vi "Read Position.vi"(8 "error in (no error)":errorcluster, 11 "Stage Actor.lvlib:Stage.lvclass":refnum<class "Stage.lvclass">) -> (0 "error out":errorcluster, 3 "Stage Actor.lvlib:Stage.lvclass":refnum<class "Stage.lvclass">)   [LabVIEW 2018, in "Stage Actor.lvlib" / "Stage.lvclass"]
uses:
  Stage.lvclass
  Stage.lvclass/Stage.ctl
  <instrlib>/Zaber A Series/Zaber A Series.lvlib
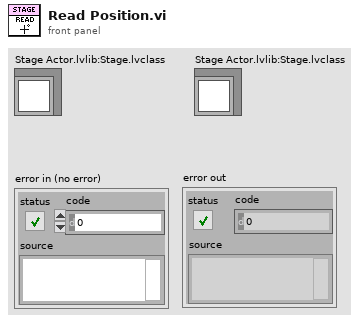
[diagram p1: front panel]
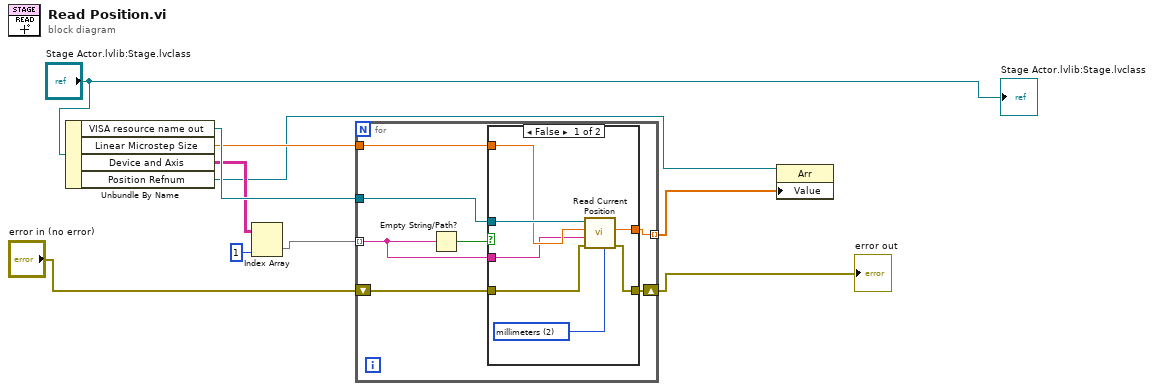
[diagram p0: block diagram]
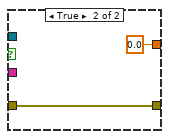
[diagram p2: hidden frame]
diagram:
  n1 = Unbundle By Name("Stage Actor.lvlib:Stage.lvclass") -> ("VISA resource name out"=w10:refnum<visa-resource-name>, "Linear Microstep Size"=w7:dbl, "Device and Axis"=w6:string[][], "Position Refnum"=w3:refnum<vi>)
  n2 = Index Array(array=w6, index (col)=1 ("disabled index (col)")) -> (element=w4:string[])  [unwired: 1 in]
  n3 = for {
    shift-right: [w16] -> w8
    shift-left: "error in (no error)" -> [w17]
    tunnel: [w14] -> w2 mode=indexing
    tunnel: w10 -> [w15]
    tunnel: w7 -> [w13]
    tunnel: w4 -> [w11] mode=indexing
    n4 = Empty String/Path?(string/path=w11) -> (empty?=w12:bool)
    n5 = case shown="False" w12 {
      tunnel: w17 -> [w24 w25]
      tunnel: [w23 w25] -> w16
      tunnel: w15 -> [w21 _]
      tunnel: [w20 0.0 ("Position")] -> w14
      tunnel: w13 -> [w19 _]
      tunnel: w11 -> [w18 _]
      frame False {
        w22 = u16 2 items=["microsteps", "microns", "millimeters", "inches", "degrees"] ("Units (0: microsteps)")
        n6 = call <instrlib>:"Read Current Position.vi"("Units (0: microsteps)"=w22, "error in (no error)"=w24, "Device and Axis"=w18, "Microstep Size (0)"=w19, "VISA resource name"=w21) -> ("error out"=w23:errorcluster, "Position"=w20:dbl)  [unwired: 4 in, 1 out]
      }
      frame True {
      }
    }
  }
  "error out" <- w8
  n7 = property class="Arr"(reference=w3, "Value"=w2) -> ()  [unwired: 1 in, 2 out]
  "Stage Actor.lvlib:Stage.lvclass" <- "Stage Actor.lvlib:Stage.lvclass"
